vi "CRYReplace CurveLib by Hardware.vi"(8 "New Name":string, 9 "Old Name":string, 10 "Type In":enum16{"Add", "Delete", "Rename"}(ring), 11 "Is Input?":bool) -> ()   [LabVIEW 2013]
uses:
  CRYProject Editor Global.vi
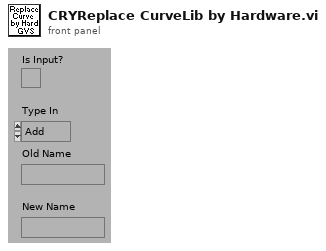
[diagram p1: front panel]
types:
  T1 = typedef "CRYTS.ctl" = cluster{"No.TS":u16, "TS File Path":path, "TS Name":string, "EditStepName":string, "Steps":T2[], "New State":bool, "Change State":bool, "Flattened CurveLib Data":string, "Document Data":string, "EditStepNo":u16, "Operator Start File":string, "Sequence Type":string, "Sequence Language":string}
  T2 = typedef "CRYStep.ctl" = cluster{"No.VI":i32, "Category":string, "StepName":string, "Seq setup flattened":string, "Comment":string, "Steps config.":bool[], "Jump config":i32[], "Start":dbl, "Increment":dbl, "Name":string, "Unit":string, "Y data":u16, "Y prefix":string, "Y dB ref":dbl, "Y unit":string, "Repeat State Array":cluster{"Start":dbl, "Increment":dbl, "Count":i32, "Num":i32}[]}
  T3 = typedef "CRYAcquisition Cluster.ctl" = cluster{"Mode":u16, "Name":string, "use ch name":bool, "Record Time":dbl, "hide rec":bool, "hide play":bool, "rec delay":dbl, "rec pad":dbl, "dcc units":i8, "sine gen setting":string, "scope_fft setting":string, "voltmeter setting":string, "rta setting":string, "trig offset(sec)":dbl, "triggered  record":bool, "trig level":dbl, "trig unit":u8, "trig slop":bool, "trig timeout(sec)":dbl, "add record":bool, "EQ":bool, "record table":string[][], "play table":string[][], "trig channel":string, "Help":string}
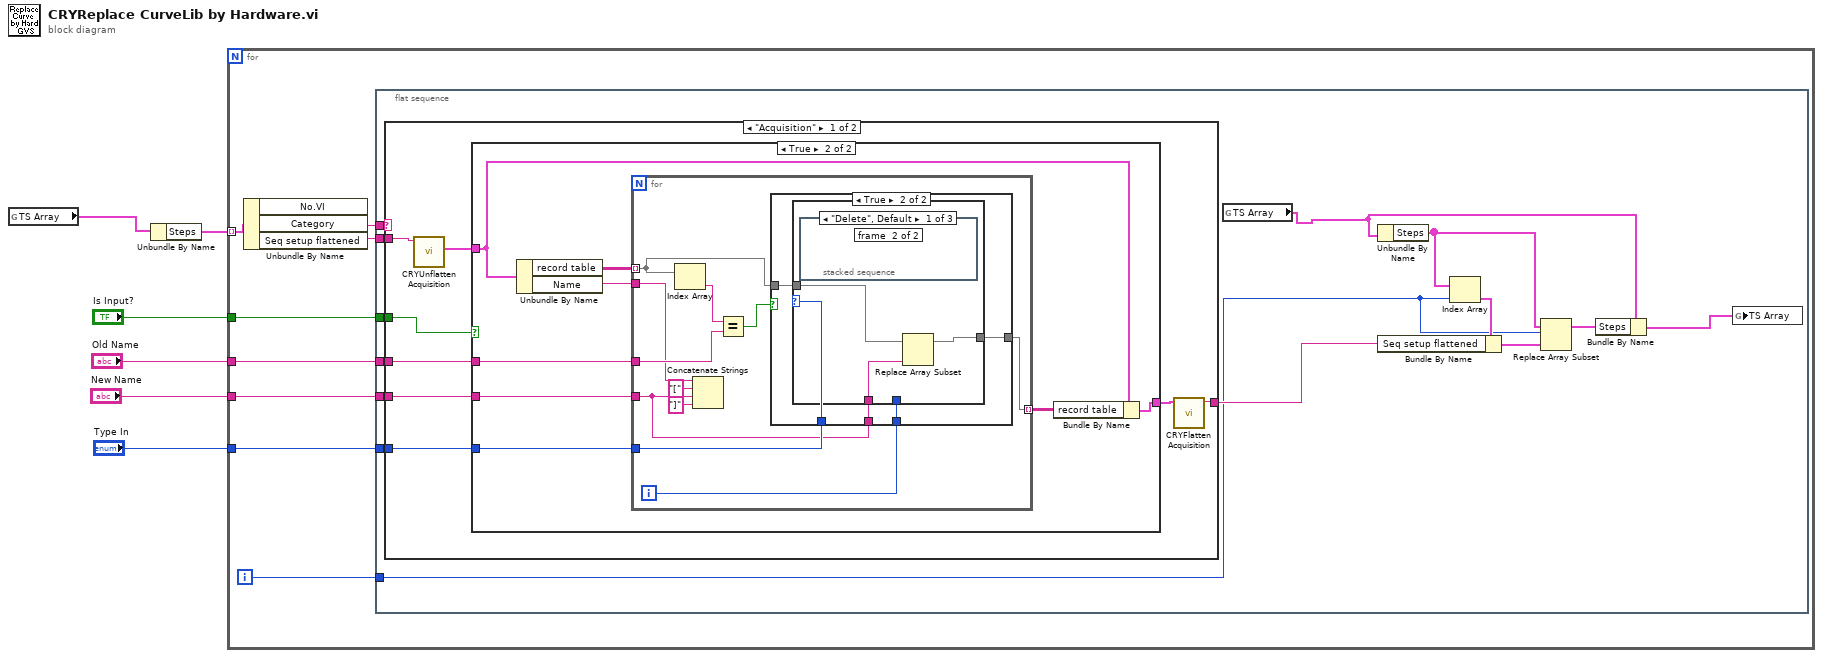
[diagram p0: block diagram]
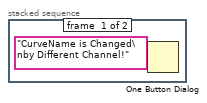
[diagram p4: hidden frame]
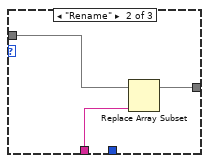
[diagram p5: hidden frame]
diagram:
  n1 = global read "CRYProject Editor Global.vi" "TS Array"() -> (w1:T1)
  n2 = Unbundle By Name(w1) -> ("Steps"=w6:T2[])
  n3 = for {
    tunnel: w6 -> [w14] mode=indexing
    tunnel: "Is Input?" -> [w11]
    tunnel: "Old Name" -> [w10]
    tunnel: "Type In" -> [w9]
    tunnel: "New Name" -> [w8]
    i -> [w7]
    n4 = Unbundle By Name(w14) -> ("Category"=w13:string, "Seq setup flattened"=w12:string)  [unwired: 1 out]
    n5 = flat-sequence {
      tunnel: w7 -> [w17]
      tunnel: w8 -> [w23]
      tunnel: w9 -> [w24]
      tunnel: w10 -> [w25]
      tunnel: w11 -> [w26]
      tunnel: w12 -> [w27]
      tunnel: w13 -> [w28]
      frame #0 {
        n6 = case shown="\"Acquisition\"" w28 {
          tunnel: w27 -> [w32 w71]
          tunnel: w26 -> [w36 _]
          tunnel: w25 -> [w35 _]
          tunnel: w24 -> [w34 _]
          tunnel: w23 -> [w33 _]
          tunnel: [w30 w71] -> w21
          frame "Acquisition" {
            n7 = call "CRYUnflatten Acquisition.vi"("Flatten Acquisition"=w32) -> ("Acquisition"=w31:T3)  [unwired: 10 out]
            n8 = case shown="True" w36 {
              tunnel: w35 -> [_ w44]
              tunnel: w34 -> [_ w43]
              tunnel: w33 -> [_ w41]
              tunnel: w31 -> [w37 w39]
              tunnel: [w37 w38] -> w29
              frame False {
              }
              frame True {
                n9 = Unbundle By Name(w39) -> ("record table"=w45:string[][], "Name"=w42:string)
                n10 = for {
                  tunnel: w45 -> [w49] mode=indexing
                  tunnel: w44 -> [w56]
                  tunnel: w43 -> [w54]
                  tunnel: w42 -> [w53]
                  tunnel: w41 -> [w48]
                  tunnel: [w46] -> w40 mode=indexing
                  i -> [w47]
                  n11 = Index Array(array=w49) -> (element=w50:string)  [unwired: 1 in]
                  n12 = Concatenate Strings(w53, "[" ("string"), w48, "]" ("string")) -> ()  [unwired: 1 out]
                  n13 = Equal?(x=w50, y=w56) -> (x = y?=w55:bool)
                  n14 = case shown="True" w55 {
                    tunnel: w54 -> [_ w62]
                    tunnel: w49 -> [w57 w61]
                    tunnel: w48 -> [_ w60]
                    tunnel: [w57 w59] -> w46
                    tunnel: w47 -> [_ w58]
                    frame False {
                    }
                    frame True {
                      n15 = case shown="\"Delete\", Default" w62 {
                        tunnel: w61 -> [w65 w69 w70]
                        tunnel: w60 -> [w64 w68 _]
                        tunnel: [w63 w67 w70] -> w59
                        tunnel: w58 -> [_ _ _]
                        frame "Delete", Default {
                          n16 = stacked-sequence {
                            frame #0 {
                              n17 = One Button Dialog(message="CurveName is Changed\nby Different Channel!") -> ()  [unwired: 2 out]
                            }
                            frame #1 {
                            }
                          }
                          n18 = Replace Array Subset(array=w65, new element=w64) -> (w63:string[])  [unwired: 1 in]
                        }
                        frame "Rename" {
                          n19 = Replace Array Subset(array=w69, new element=w68) -> (w67:string[])  [unwired: 1 in]
                        }
                        frame "Add" {
                        }
                      }
                    }
                  }
                }
                n20 = Bundle By Name(cluster=w39, "record table"=w40) -> (w38:T3)
              }
            }
            n21 = call "CRYFlatten Acquisition.vi"("Acquisition"=w29) -> ("Acquisition flattened"=w30:string)  [unwired: 10 out]
          }
          frame "Calibration", Default {
          }
        }
        n22 = global read "CRYProject Editor Global.vi" "TS Array"() -> (w16:T1)
        n23 = Unbundle By Name(w16) -> ("Steps"=w20:T2[])
        n24 = Index Array(array=w20, index=w17) -> (element=w22:T2)
        n25 = Bundle By Name(cluster=w22, "Seq setup flattened"=w21) -> (w19:T2)
        n26 = Replace Array Subset(array=w20, new element=w19, index=w17) -> (w18:T2[])
        n27 = Bundle By Name(cluster=w16, "Steps"=w18) -> (w15:T1)
        n28 = global write "CRYProject Editor Global.vi" "TS Array"(w15) -> ()
      }
    }
  }
